vi "exp5.vi"() -> ()   [LabVIEW 2019]
uses:
  <vilib>/Analysis/Matrix/Datatypes/RealMatrix.ctl
  <vilib>/Analysis/2dsp.llb/Real FFT.vi
  <vilib>/Analysis/baseanly.llb/Mean (DBL).vi
  <vilib>/Analysis/2dsp.llb/1D Auto Correlation (DBL).vi
  <vilib>/Analysis/3filter.llb/IIR Filter (DBL).vi
  <vilib>/Analysis/7linalg.llb/Create Special Real Matrix.vi
  <vilib>/Analysis/baseanly.llb/Real Inverse Matrix.vi
  <vilib>/Analysis/3filter.llb/FIR Filter (DBL).vi
  <vilib>/Analysis/2dsp.llb/1D Cross Correlation (DBL).vi
  <vilib>/Analysis/BLAS.llb/dgemv - General Matrix-Vector Product (DBL).vi
  <vilib>/Analysis/Matrix/Numeric/Multiply/Multiply - RM,R.vi
  <vilib>/Analysis/Matrix/Numeric/Add/Add - RM,RM.vi
  <vilib>/Analysis/NI_AALBase.lvlib
  <vilib>/Analysis/NI_AALBLAS.lvlib
  <vilib>/Analysis/NI_AALPro.lvlib
  <vilib>/Analysis/Matrix/NI_Matrix.lvlib
panel:
  out "old":dbl
  in  "innovation standard deviation":dbl=1.0000000000000002 format="%0.2f"
  out "Rdx":dbl[](array[numeric])
  out "PM Filter Frequency Response":dbl[](graph)
  out "Wiener Filter Frequency Response":dbl[](graph)
  out "Wiener Filter Error, PM Filter Error":waveform(dbl)[](graph)
  out "Input, Wiener Filter Output, PM Filter Output":waveform(dbl)[](graph)
  in  "stop":bool
  out "MSE Wiener Filter":dbl
  out "LSE Parks Mccellan Filter":dbl format="%0.2f"
  out "LSE Wiener Filter":dbl format="%0.2f"
  out "FIR Wiener Filter Coefficients":dbl[](array[numeric])
  out "Rx Matrix":T1
  in  "Pstep":i32
  in  "FIR Wiener Filter Length":i32
  in  "# of taps":i32=32
  in  "Band Parameters for Parks Mccellan Filter":T2(array[cluster])=[{"Amplitude"=1.0, "Lower Freq"=0.0, "Higher Freq"=0.2, "Weighted\nRipple"=1.0}, {"Amplitude"=0.0, "Lower Freq"=0.25, "Higher Freq"=0.5, "Weighted\nRipple"=1.0}] {"Weighted\nRipple" min=-1e-308 max=1e+308 format="%0.2e"; "Higher Freq" min=-1e-308 max=1e+308 format="%0.2f"; "Lower Freq" min=-1e-308 max=1e+308 format="%0.2f"; "Amplitude" min=-1e-308 max=1e+308 format="%0.2f"}
  in  "environment standard deviation":dbl=1.0000000000000002 format="%0.2f"
  in  "innovations process pole":dbl
  in  "samples":i32=128
  in  "millisecond timer value":u32
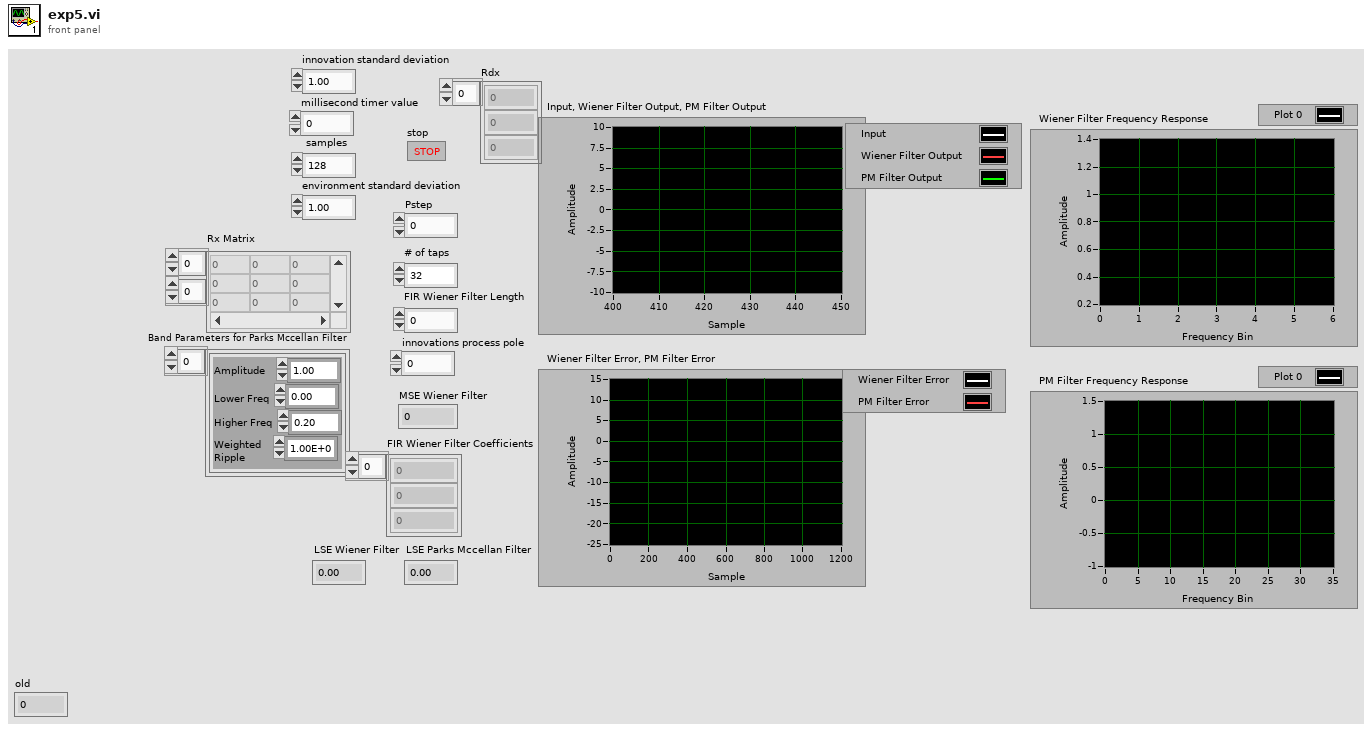
[diagram p1: front panel]
types:
  T1 = typedef "NI_Matrix.lvlib/RealMatrix.ctl" = dbl[][]
  T2 = cluster{"Amplitude":dbl, "Lower Freq":dbl, "Higher Freq":dbl, "Weighted\nRipple":dbl}[]
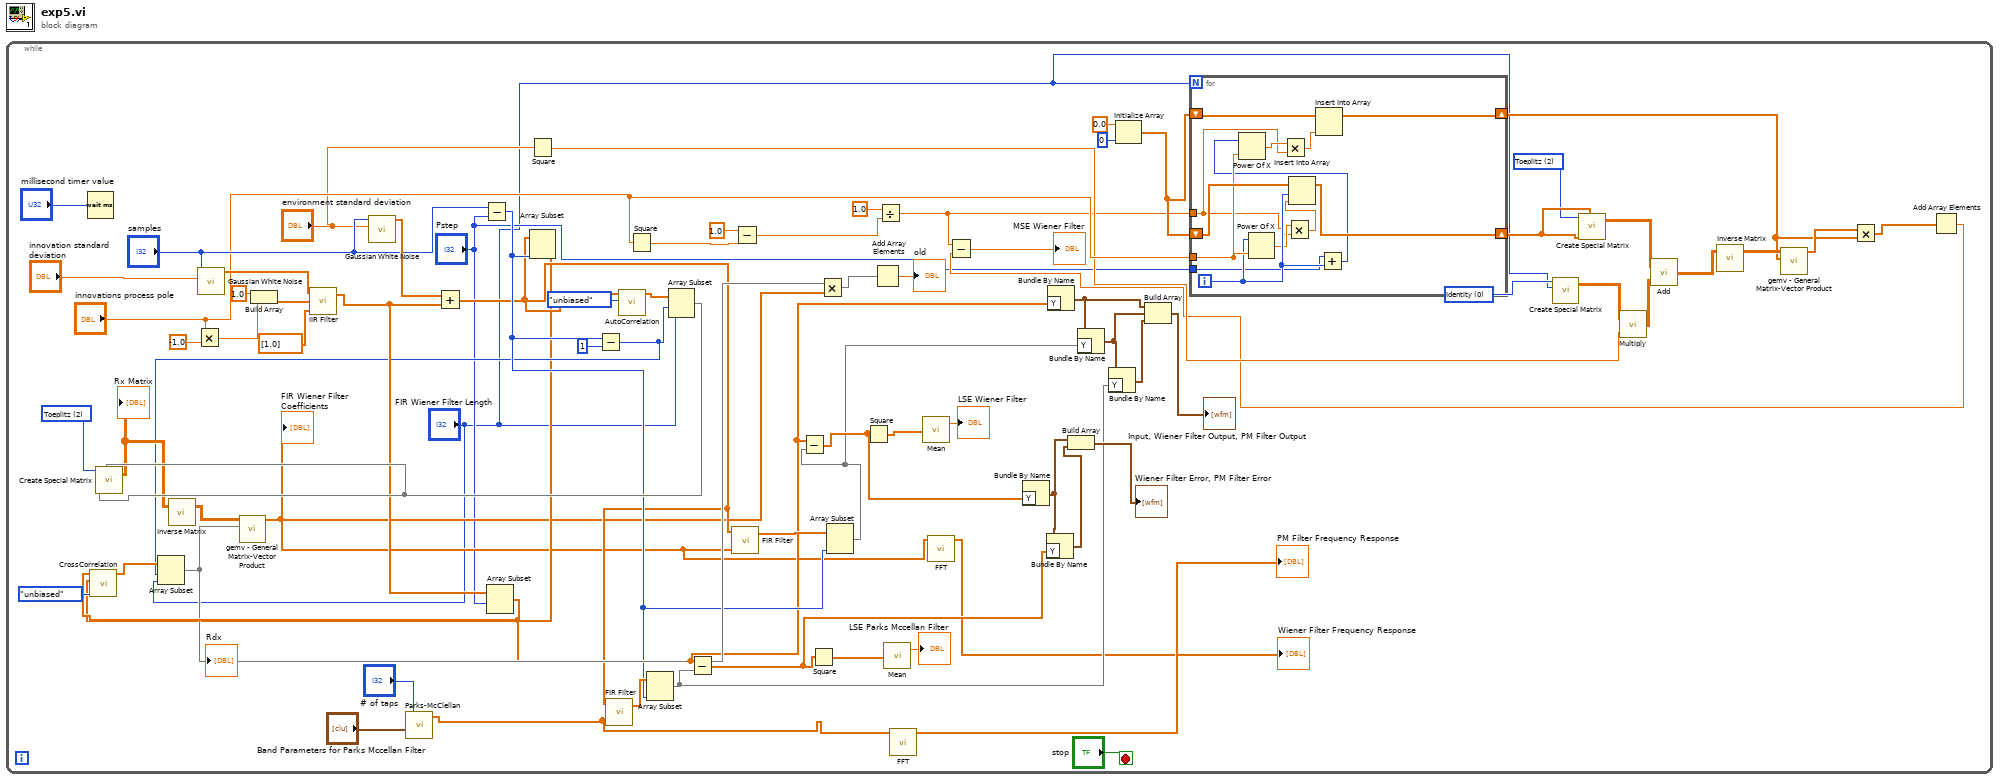
[diagram p0: block diagram]
diagram:
  n1 = while {
    stop <- "stop" stop-if-true
    w19 = 0 items=["Identity", "Diagonal", "Toeplitz", "Vandermonde", "Companion", "Hankel", "Hadamard", "Wilkinson", "Hilbert", "Inverse Hilbert", "Rosser", "Pascal"] ("matrix type")
    w20 = 2 items=["Identity", "Diagonal", "Toeplitz", "Vandermonde", "Companion", "Hankel", "Hadamard", "Wilkinson", "Hilbert", "Inverse Hilbert", "Rosser", "Pascal"] ("matrix type")
    w69 = 2 items=["Identity", "Diagonal", "Toeplitz", "Vandermonde", "Companion", "Hankel", "Hadamard", "Wilkinson", "Hilbert", "Inverse Hilbert", "Rosser", "Pascal"] ("matrix type")
    n2 = Wait (ms)(milliseconds to wait="millisecond timer value") -> ()  [unwired: 1 out]
    n3 = Multiply(x="innovations process pole", y=-1.0) -> (x*y=w73:dbl)
    n4 = call <vilib>:"Gaussian White Noise.vi"("standard deviation"="innovation standard deviation", "samples"="samples") -> ("Gaussian noise pattern"=w77:dbl[])  [unwired: 8 in, 1 out]
    n5 = Build Array(1.0 ("element"), w73) -> (w75:dbl[])
    n6 = call-poly <vilib>:"IIR Filter.vi"("Forward Coefficients"=dbl[] [1.0], "Reverse Coefficients"=w75, "X"=w77) -> ("Filtered X"=w57:dbl[])  [unwired: 1 in, 1 out]
    n7 = call <vilib>:"Gaussian White Noise.vi"("standard deviation"="environment standard deviation", "samples"="samples") -> ("Gaussian noise pattern"=w72:dbl[])  [unwired: 8 in, 1 out]
    n8 = call <vilib>:"Parks-McClellan.vi"("Band Parameters"="Band Parameters for Parks Mccellan Filter", "# of taps"="# of taps") -> ("h"=w28:dbl[])  [unwired: 2 in, 2 out]
    n9 = Add(x=w72, y=w57) -> (x+y=w36:dbl[])
    n10 = Subtract(x="samples", y="Pstep") -> (x-y=w44:i32)
    n11 = Array Subset(array=w57, index="Pstep") -> (w64:dbl[])  [unwired: 1 in]
    n12 = Square(x="environment standard deviation") -> (x^2=w17:dbl)
    n13 = Array Subset(array=w36, length=w44) -> (w29:dbl[])  [unwired: 1 in]
    n14 = call-poly <vilib>:"CrossCorrelation.vi"("normalization"=enum32{"none", "unbiased", "biased"}."unbiased", "Y"=w29, "X"=w64) -> ("Rxy"=w61:dbl[])  [unwired: 7 in, 1 out]
    n15 = Subtract(x=w44, y=1) -> (x-y=w42:i32)
    n16 = Array Subset(array=w61, index=w42, length="FIR Wiener Filter Length") -> (w48:dbl[])
    "Rdx" <- w48
    n17 = call-poly <vilib>:"FIR Filter.vi"("FIR Coefficients"=w28, "X"=w36) -> ("Filtered X"=w54:dbl[])  [unwired: 2 in, 1 out]
    n18 = call-poly <vilib>:"AutoCorrelation.vi"("normalization"=enum32{"none", "unbiased", "biased"}."unbiased", "X"=w36) -> ("Rxx"=w67:dbl[])  [unwired: 8 in, 1 out]
    n19 = Square(x="innovations process pole") -> (x^2=w50:dbl)
    n20 = Array Subset(array=w54, length=w44) -> (w34:dbl[])  [unwired: 1 in]
    n21 = Array Subset(array=w67, index=w42, length="FIR Wiener Filter Length") -> (w65:dbl[])
    n22 = call-poly <vilib>:"Create Special Matrix.vi"("matrix type"=w69, "Input Vector1"=w65, "Input Vector2"=w65) -> ("Special Matrix"=w60:T1)  [unwired: 2 in, 1 out]
    "Rx Matrix" <- w60
    n23 = call-poly <vilib>:"Inverse Matrix.vi"("Input Matrix"=w60) -> ("Inverse Matrix"=w68:T1)  [unwired: 1 in, 1 out]
    n24 = call-poly <vilib>:"gemv - General Matrix-Vector Product.vi"("x"=w48, "A"=w68) -> ("dgemv"=w26:dbl[])  [unwired: 8 in, 1 out]
    "FIR Wiener Filter Coefficients" <- w26
    n25 = Subtract(x=w29, y=w34) -> (x-y=w40:dbl[])
    n26 = call-poly <vilib>:"FIR Filter.vi"("FIR Coefficients"=w26, "X"=w36) -> ("Filtered X"=w53:dbl[])  [unwired: 2 in, 1 out]
    n27 = Subtract(x=1.0, y=w50) -> (x-y=w49:dbl)
    n28 = Square(x=w40) -> (x^2=w56:dbl[])
    n29 = Multiply(x=w48, y=w26) -> (x*y=w47:dbl[])
    n30 = Array Subset(array=w53, length=w44) -> (w35:dbl[])  [unwired: 1 in]
    n31 = Subtract(x=w29, y=w35) -> (x-y=w41:dbl[])
    n32 = Square(x=w41) -> (x^2=w59:dbl[])
    n33 = Add Array Elements(numeric array=w47) -> (sum=→"old":dbl)
    n34 = Divide(x=1.0, y=w49) -> (x/y=w1:dbl)
    n35 = call-poly <vilib>:"Mean.vi"("X"=w56) -> ("mean"=→"LSE Parks Mccellan Filter":dbl)  [unwired: 1 out]
    n36 = call-poly <vilib>:"FFT.vi"("X"=w28) -> ("FFT {X}"=→"PM Filter Frequency Response":cdb[])  [unwired: 9 in, 1 out]
    n37 = call-poly <vilib>:"Mean.vi"("X"=w59) -> ("mean"=→"LSE Wiener Filter":dbl)  [unwired: 1 out]
    n38 = call-poly <vilib>:"FFT.vi"("X"=w26) -> ("FFT {X}"=→"Wiener Filter Frequency Response":cdb[])  [unwired: 9 in, 1 out]
    n39 = Bundle By Name("Y"=w41) -> (w38:waveform(dbl))  [unwired: 1 in]
    n40 = Bundle By Name(cluster=w38, "Y"=w40) -> (w39:waveform(dbl))
    n41 = Bundle By Name("Y"=w29) -> (w31:waveform(dbl))  [unwired: 1 in]
    n42 = Build Array(w38, w39) -> (→"Wiener Filter Error, PM Filter Error":waveform(dbl)[])
    n43 = Bundle By Name(cluster=w31, "Y"=w35) -> (w32:waveform(dbl))
    n44 = Bundle By Name(cluster=w32, "Y"=w34) -> (w33:waveform(dbl))
    n45 = Initialize Array(0.0 ("element"), 0 ("dimension size")) -> (w2:dbl[])
    n46 = Build Array(w31, w32, w33) -> (→"Input, Wiener Filter Output, PM Filter Output":waveform(dbl)[])
    n47 = for {
      N: "FIR Wiener Filter Length" -> [_]
      shift-right: [w91] -> w21
      shift-left: w2 -> [w90]
      tunnel: "innovations process pole" -> [w87]
      shift-right: [w88] -> w9
      shift-left: w2 -> [w89]
      tunnel: "Pstep" -> [w85]
      tunnel: w1 -> [w79]
      i -> [w86]
      n48 = Power Of X(1:w87, 2:w86) -> (0:w80:dbl)
      n49 = Multiply(x=w80, y=w79) -> (x*y=w83:dbl)
      n50 = Insert Into Array(array=w90, index=w86, new element=w83) -> (w91:dbl[])
      n51 = Add(x=w85, y=w86) -> (x+y=w84:i32)
      n52 = Power Of X(1:w87, 2:w84) -> (0:w81:dbl)
      n53 = Multiply(x=w81, y=w79) -> (x*y=w82:dbl)
      n54 = Insert Into Array(array=w89, new element=w82) -> (w88:dbl[])  [unwired: 1 in]
    }
    n55 = call-poly <vilib>:"Create Special Matrix.vi"("matrix type"=w19, "matrix size"="FIR Wiener Filter Length") -> ("Special Matrix"=w16:T1)  [unwired: 3 in, 1 out]
    n56 = call-poly <vilib>:"Create Special Matrix.vi"("matrix type"=w20, "Input Vector1"=w21, "Input Vector2"=w21) -> ("Special Matrix"=w14:T1)  [unwired: 2 in, 1 out]
    n57 = call-poly <vilib>:"Multiply.vi"("Real Scalar c"=w17, "Real Matrix A"=w16) -> ("A * c"=w15:T1)
    n58 = call-poly <vilib>:"Add.vi"("Real Matrix B"=w15, "Real Matrix A"=w14) -> ("A + B"=w13:T1)
    n59 = call-poly <vilib>:"Inverse Matrix.vi"("Input Matrix"=w13) -> ("Inverse Matrix"=w12:T1)  [unwired: 1 in, 1 out]
    n60 = call-poly <vilib>:"gemv - General Matrix-Vector Product.vi"("x"=w9, "A"=w12) -> ("dgemv"=w10:dbl[])  [unwired: 8 in, 1 out]
    n61 = Multiply(x=w10, y=w9) -> (x*y=w11:dbl[])
    n62 = Add Array Elements(numeric array=w11) -> (sum=w8:dbl)
    n63 = Subtract(x=w1, y=w8) -> (x-y=→"MSE Wiener Filter":dbl)
  }
